vi "Get Element.vi"(8 "error in (no error)":errorcluster, 10 "GetElement (-1: Current)":i32=-1, 11 "CircularBuffer":refnum<class "CircularBuffer.lvclass">) -> (0 "error out":errorcluster, 2 "Element":variant, 3 "CircularBuffer out":refnum<class "CircularBuffer.lvclass">)   [LabVIEW 2013, in "CircularBuffer.lvclass"]
doc: "---------------------------------------------------------------\nJKI State Machine Objects™\nhttp://jki.net/state-machine-objects/\nCopyright (C) 2005-2015, JKI <info@jki.net>\nALL RIGHTS RESERVEDJKI State Machine Objects (SMO) 1.0.0.4\nJKI - JKI\nCopyright (c) 2015, JKI"
uses:
  CircularBuffer.lvclass
  types/type/type.lvclass
panel:
  # "For instructions on how to use the JKI State Machine Objects, examples and video tutorials, visit:\nhttp://jki.net/state-machine-objects/\n\nJKI State Machine Objects™\nhttp://jki.net/state-machine-objects/\nCopyright (C) 2005-2015, JKI <info@jki.net>\nALL RIGHTS RESERVED"
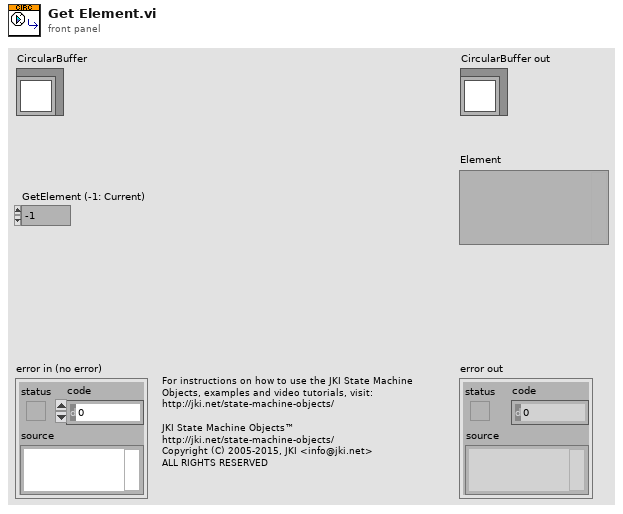
[diagram p1: front panel]
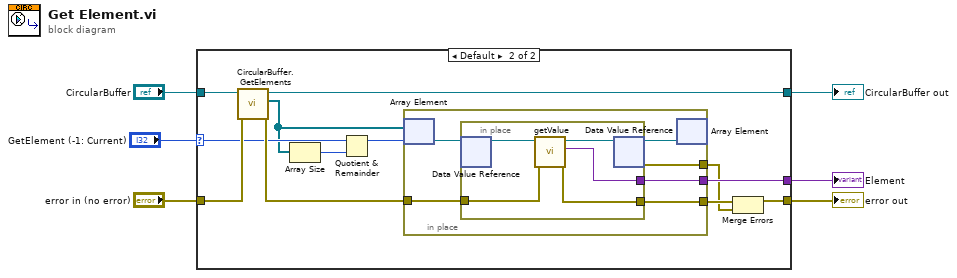
[diagram p0: block diagram]
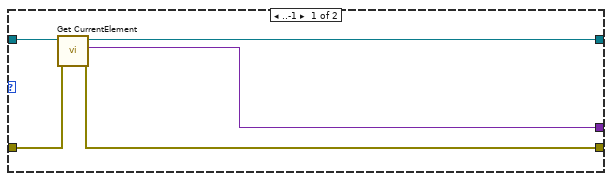
[diagram p2: hidden frame]
diagram:
  n1 = case shown="Default" "GetElement (-1: Current)" {
    selector: "GetElement (-1: Current)" -> [_ w15]
    tunnel: [w10 w23] -> w6
    tunnel: [w8 w22] -> w5
    tunnel: "error in (no error)" -> [w9 w21]
    tunnel: "CircularBuffer" -> [w11 w20]
    tunnel: [w7 w19] -> w2
    frame ..-1 {
      n2 = call "Get CurrentElement.vi"("error in (no error)"=w9, "CircularBuffer"=w11) -> ("error out"=w8:errorcluster, "Element"=w7:variant, "CircularBuffer out"=w10:refnum<class "CircularBuffer.lvclass">)  [unwired: 7 in]
    }
    frame Default {
      n3 = call "CircularBuffer.GetElements.vi"("error in (no error)"=w21, "CircularBuffer in"=w20) -> ("error out"=w18:errorcluster, "Elements"=w13:refnum<data-value>[], "CircularBuffer out"=w23:refnum<class "CircularBuffer.lvclass">)  [unwired: 7 in]
      n4 = Array Size(array=w13) -> (size(s)=w12:i32)
      n5 = Quotient & Remainder(x=w15, y=w12) -> (x-y*floor(x/y)=w14:i32)  [unwired: 1 out]
      n6 = in-place {
        in-place-border: [w29] -> w19
        in-place-border: w18 -> [w28]
        in-place-border: [w27] -> w17
        in-place-border: [w26] -> w16
        n7 = in-place-array #1(w13, w14) -> (w25:refnum<data-value>)
        n8 = in-place {
          in-place-border: [w32] -> w29
          in-place-border: w28 -> [w31]
          in-place-border: [w30] -> w27
          n9 = in-place-dvr #2(w25) -> (w34:refnum<class "type.lvclass">)  [unwired: 1 out]
          n10 = call-dynamic "getValue.vi"("error in (no error)"=w31, "type in"=w34) -> ("error out"=w30:errorcluster, "value"=w32:variant, "type out"=w33:refnum<class "type.lvclass">)  [unwired: 7 in]
          n11 = in-place-dvr #2(w33) -> (w24:refnum<data-value>, w26:errorcluster)
        }
        n12 = in-place-array #1(w24) -> ()  [unwired: 2 out]
      }
      n13 = Merge Errors(w17, w16) -> (w22:errorcluster)
    }
  }
  "error out" <- w5
  "CircularBuffer out" <- w6
  "Element" <- w2
